vi "Inline - Monitor Sequential Monitor.vi"(8 "error in (no error)":errorcluster, 11 "core handle in":u64) -> (0 "error out":errorcluster, 3 "core handle out":u64)   [LabVIEW 2019, in "Ballard Arinc-429 Engine.lvlib"]
uses:
  Ballard Arinc-429 Engine.lvlib
  <instrlib>/BTICardLib/BTICardLV.lvlib
  <vilib>/NI VeriStand/Custom Device Tools/Custom Device Utility Library/Custom Device Utility Library.lvlib
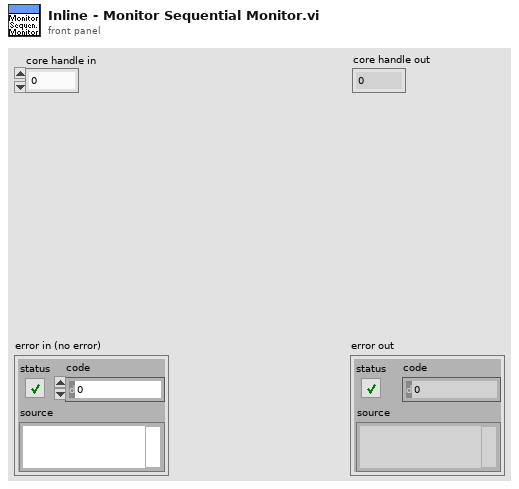
[diagram p1: front panel]
types:
  T1 = typedef "BTICardLV.lvlib/Seq Run Status.ctl" = u32
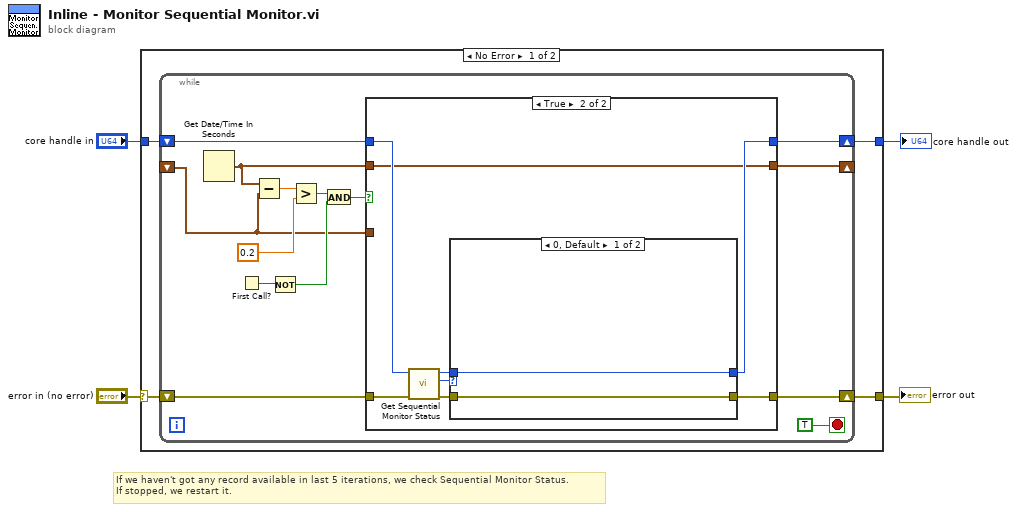
[diagram p0: block diagram]
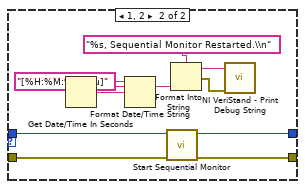
[diagram p3: hidden frame]
diagram:
  # "If we haven't got any record available in last 5 iterations, we check Sequential Monitor Status.\nIf stopped, we restart it."
  n1 = case shown="No Error" "error in (no error)" {
    selector: "error in (no error)" -> [w8 w47]
    tunnel: [w7 w47] -> w3
    tunnel: "core handle in" -> [w6 w46]
    tunnel: [w5 w46] -> w1
    frame No Error {
      n2 = while {
        shift-right: [w21] -> w7
        shift-left: w8 -> [w22]
        shift-right: [w19] -> w5
        shift-left: w6 -> [w20]
        shift-right: [w9] -> _
        shift-left: _ -> [w11]
        stop <- TRUE stop-if-true
        n3 = Get Date/Time In Seconds() -> (seconds since 1Jan1904=w10:timestamp)
        n4 = First Call?() -> (First Call?: T/F=w14:bool)
        n5 = Subtract(x=w10, y=w11) -> (x-y=w17:dbl)
        n6 = Not(x=w14) -> (.not. x?=w13:bool)
        n7 = Greater?(x=w17, y=0.2) -> (0:w15:bool)
        n8 = And(x=w15, y=w13) -> (x .and. y?=w12:bool)
        n9 = case shown="True" w12 {
          tunnel: w22 -> [w25 w33]
          tunnel: [w25 w27] -> w21
          tunnel: w20 -> [w23 w32]
          tunnel: [w23 w29] -> w19
          tunnel: w11 -> [w24 _]
          tunnel: [w24 w26] -> w9
          tunnel: w10 -> [_ w26]
          frame False {
          }
          frame True {
            n10 = call <instrlib>:"Get Sequential Monitor Status.vi"("error in (no error)"=w33, "core handle in"=w32) -> ("error out"=w28:errorcluster, "run status"=w31:T1, "core handle out"=w30:u64)  [unwired: 6 in, 1 out]
            n11 = case shown="0, Default" w31 {
              tunnel: w30 -> [w35 w45]
              tunnel: [w35 w42] -> w29
              tunnel: w28 -> [w34 w44]
              tunnel: [w34 w43] -> w27
              frame 0, Default {
              }
              frame 1, 2 {
                n12 = Get Date/Time In Seconds() -> (seconds since 1Jan1904=w36:timestamp)
                n13 = Format Date/Time String(time format string (%c)="[%H:%M:%S%3u]", seconds (now)=w36) -> (date/time string=w37:string)  [unwired: 1 in]
                n14 = call <instrlib>:"Start Sequential Monitor.vi"("error in (no error)"=w44, "core handle in"=w45) -> ("error out"=w43:errorcluster, "core handle out"=w42:u64)  [unwired: 8 in]
                n15 = Format Into String(format string="%s, Sequential Monitor Restarted.\\n", w37) -> (resulting string=w41:string, error out=w40:errorcluster)  [unwired: 2 in]
                n16 = call <vilib>:"NI VeriStand - Print Debug String.vi"("error in (no error)"=w40, "Message"=w41) -> ()  [unwired: 9 in, 1 out]
              }
            }
          }
        }
      }
    }
    frame Error {
    }
  }
  "error out" <- w3
  "core handle out" <- w1
